vi "Read Value.vi"(8 "error in (no error)":errorcluster caption="entrée d'erreur (pas d'erreur)", 11 "DAQmxTaskCounterDigital en entrée":refnum<class "DAQmxTaskCounterDigital.lvclass">) -> (0 "error out":errorcluster caption="sortie d'erreur", 1 "Data":bool, 2 "Data string":string, 3 "DAQmxTaskCounterDigital en sortie":refnum<class "DAQmxTaskCounterDigital.lvclass">)   [LabVIEW 2015, in "DAQmxTaskCounterDigital.lvclass"]
uses:
  DAQmxTaskCounterDigital.lvclass
  DAQmxTask.lvclass/DAQmxTask.ctl
  <vilib>/DAQmx/read.llb/DAQmx Read (Counter DBL 1Chan 1Samp).vi
  <vilib>/DAQmx/miscellaneous.llb/DAQmx Fill In Error Info.vi
  DAQmxTask.lvclass
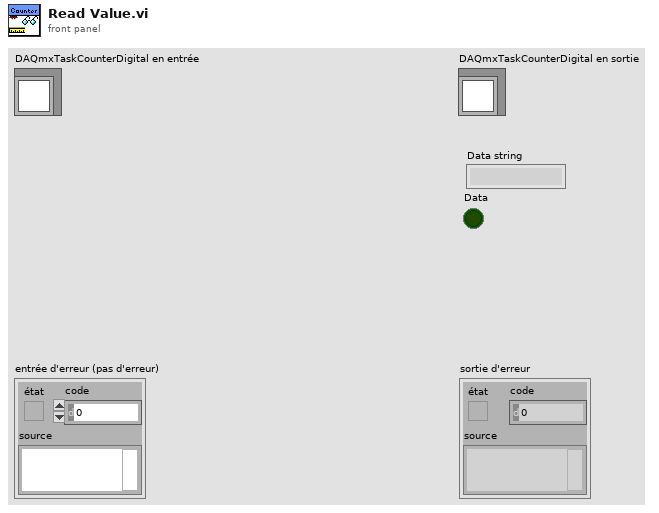
[diagram p1: front panel]
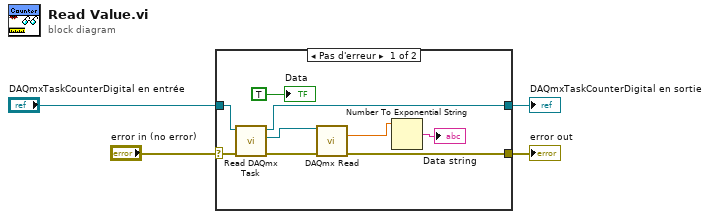
[diagram p0: block diagram]
diagram:
  n1 = case shown="Pas d'erreur" "error in (no error)" {
    selector: "error in (no error)" -> [w13 w15]
    tunnel: [w5 w15] -> w2
    tunnel: "DAQmxTaskCounterDigital en entrée" -> [w12 w14]
    tunnel: [w6 w14] -> w1
    frame No Error {
      n2 = call "Read DAQmx Task.vi"("error in (no error)"=w13, "DAQmxTask in"=w12) -> ("error out"=w10:errorcluster, "DAQmx Task Name"=w11:refnum<k21>, "DAQmxTask out"=w6:refnum<class "DAQmxTaskCounterDigital.lvclass">)  [unwired: 7 in]
      n3 = call-poly <vilib>:"DAQmx Read.vi"("task/channels in"=w11, "error in"=w10) -> ("data"=w9:dbl, "error out"=w5:errorcluster)  [unwired: 11 in, 1 out]
      n4 = Number To Exponential String(number=w9) -> (E-format string=→"Data string":string)  [unwired: 3 in]
      "Data" <- TRUE
    }
    frame Error {
    }
  }
  "error out" <- w2
  "DAQmxTaskCounterDigital en sortie" <- w1
